vi "Verify Scroll.vi"(0 "GEA2 Reference In":refnum<k24>, 1 "Timeout (sec)":dbl, 2 "Scroll Text":string, 11 "Error In":errorcluster, 13 "Ignore Brightness?":bool) -> (4 "GEA2 Reference Out":refnum<k24>, 6 "Pass/Fail?":bool, 8 "Report Text":string, 15 "Error Out":errorcluster)   [LabVIEW 2016, in "TLMB.lvlib"]
doc: "This VI is used to verify SSD scrolling messages on the HEUI."
uses:
  Projects/TLMB.lvlib
  Q:/Common/DLLs/GEA3/GeaCommunication.dll
  Common/DLLs/GEA3/GeaCommunication.dll
  Common/LabVIEW GEA2 Toolkit/LabVIEW_GEA2_Toolkit.lvlibp/type defs/Source_Destination.ctl
  Common/LabVIEW GEA2 Toolkit/LabVIEW_GEA2_Toolkit.lvlibp/type defs/ERD Read Data In.ctl
  Common/LabVIEW GEA2 Toolkit/LabVIEW_GEA2_Toolkit.lvlibp/type defs/Data Type.ctl
  Common/LabVIEW GEA2 Toolkit/LabVIEW_GEA2_Toolkit.lvlibp
panel:
  in  "Standalone":bool
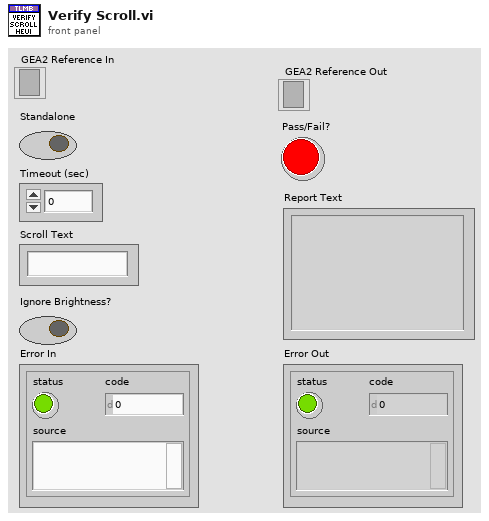
[diagram p1: front panel]
types:
  T1 = typedef "LabVIEW_GEA2_Toolkit.lvlibp/ERD Read Data In.ctl" = cluster{"ERD Number":u16, "Data Type":T2}
  T2 = typedef "LabVIEW_GEA2_Toolkit.lvlibp/Data Type.ctl" = enum16{"string", "boolean", "uint8_t", "uint16_t", "uint32_t", "uint64_t", "int8_t", "int16_t", "int32_t", "int64_t"}
  T3 = typedef "LabVIEW_GEA2_Toolkit.lvlibp/Source_Destination.ctl" = cluster{"Source":u8, "Destination":u8}
  T4 = typedef "TLMB.lvlib/HEUI_LEDs.ctl" = cluster{"Z101 - Start":bool, "Z103 - Colors":bool, "Z104 - Whites":bool, "Z105 - Towels":bool, "Z106 - Bulky Items":bool, "Z107 - Heavy Duty":bool, "Z108 - Jeans":bool, "Z109 - Basket Clean":bool, "Z110 - Drain and Spin":bool, "Z111 - Rinse and Spin":bool, "Z112 - Speed Wash":bool, "Z113 - Active Wear":bool, "Z114 - Hand Wash":bool, "Z115 - Delicates":bool, "Z116 - Easy Care":bool, "Z117 - Tomato":bool, "Z118 - Wine":bool, "Z119 - Blood":bool, "Z120 - Grass":bool, "Z121 - Dirt":bool, "Z122_MSB_A":bool, "Z123_MSB_B":bool, "Z124_MSB_G":bool, "Z125_MSB_C":bool, "Z126_MSB_D":bool, "Z127_MSB_E":bool, "Z128_MSB_F":bool, "Z129_LSB_A":bool, "Z130_LSB_B":bool, "Z131_LSB_G":bool, "Z132_LSB_C":bool, "Z133_LSB_D":bool, "Z134_LSB_E":bool, "Z135_LSB_F":bool, "Z136 - Pause":bool, "Z137 - Pause":bool, "Z138 - Lock Controls":bool, "Z139 - Lock Controls":bool, "Z140 - Lock Controls":bool, "Z141 - Lid Lock":bool, "Z142 - Lid Lock":bool, "Z143 - Lid Lock":bool, "Z144 - Good":bool, "Z145":bool, "Z146":bool, "Z147 - Better":bool, "Z148 - Delay":bool, "Z149 - Fill":bool, "Z150 - Soak":bool, "Z151 - Wash":bool, "Z152 - Rinse":bool, "Z153 - Spin":bool, "Z154 - Hot":bool, "Z155 - Warm":bool, "Z156 - Colors":bool, "Z157 - Cool":bool, "Z158 - Cold":bool, "Z159 - Tap Cold":bool, "Z160 - Extra Heavy":bool, "Z161 - Heavy":bool, "Z162 - Normal":bool, "Z163 - Light":bool, "Z164 - Max Spin":bool, "Z165 - More Spin":bool, "Z166 - Normal Spin":bool, "Z167 - No Spin":bool, "Z168 - Extra Rinse":bool, "Z170 - Deep Rinse":bool, "Z171 - Auto Soak":bool, "Z172 - Warm Rinse":bool, "Z173 - Deep Fill":bool, "Z174 - My Cycles":bool, "Z175 - Delay Wash":bool, "Z176 - Spin Stop":bool, "Z177 - Spin Stop":bool, "Z178 - Spin Stop":bool, "Z179 - Pause":bool, "Z109":bool, "Z110":bool, "Z123":bool, "Z124":bool, "Z140":bool, "Unused0":bool, "Unused1":bool, "Unused2":bool, "Unused3":bool, "Channel_Off":bool, "Channel_Cycle_Unmapped":bool}
  T5 = typedef "TLMB.lvlib/HEUI_Display.ctl" = cluster{"SSD":string, "Cycle Selection":T6, "Stain Selection":T7, "Temp Level":T8, "Soil Level":T9, "Spin Level":T10, "750 Status":T11, "Start":bool, "Pause/WiFi":bool, "Lock Controls":bool, "Lid Lock":bool, "Extra Rinse":bool, "Deep Rinse":bool, "Auto Soak":bool, "Warm Rinse":bool, "Deep Fill":bool, "My Cycle":bool, "Delay Wash":bool, "Spin Stop":bool, "Delay":bool, "Fill":bool, "Soak":bool, "Wash":bool, "Rinse":bool, "Spin":bool}
  T6 = typedef "TLMB.lvlib/Cycle Selection Enum.ctl" = enum16{"Colors", "Easy Care", "Delicates", "Hand Wash", "Active Wear", "Speed Wash", "Rinse and Spin", "Drain and Spin", "Basket Clean", "Jeans", "Heavy Duty", "Bulky Items", "Towels", "Whites", "Off", "*Incorrect*"}
  T7 = typedef "TLMB.lvlib/Stain Enum.ctl" = enum16{"Tomato", "Wine", "Blood", "Grass", "Dirt", "Off", "*Incorrect*"}
  T8 = typedef "TLMB.lvlib/Temp Enum.ctl" = enum16{"Hot", "Warm", "Colors", "Cool", "Cold", "Tap Cold", "Off", "*Incorrect*"}
  T9 = typedef "TLMB.lvlib/Soil Enum.ctl" = enum16{"Extra Heavy", "Heavy", "Normal", "Light", "Off", "*Incorrect*"}
  T10 = typedef "TLMB.lvlib/Spin Enum.ctl" = enum16{"Max Spin", "More Spin", "Normal Spin", "No Spin", "Off", "*Incorrect*"}
  T11 = typedef "TLMB.lvlib/750 Status Enum.ctl" = enum16{"Fill", "Wash", "Rinse", "Spin", "Off", "*Incorrect*"}
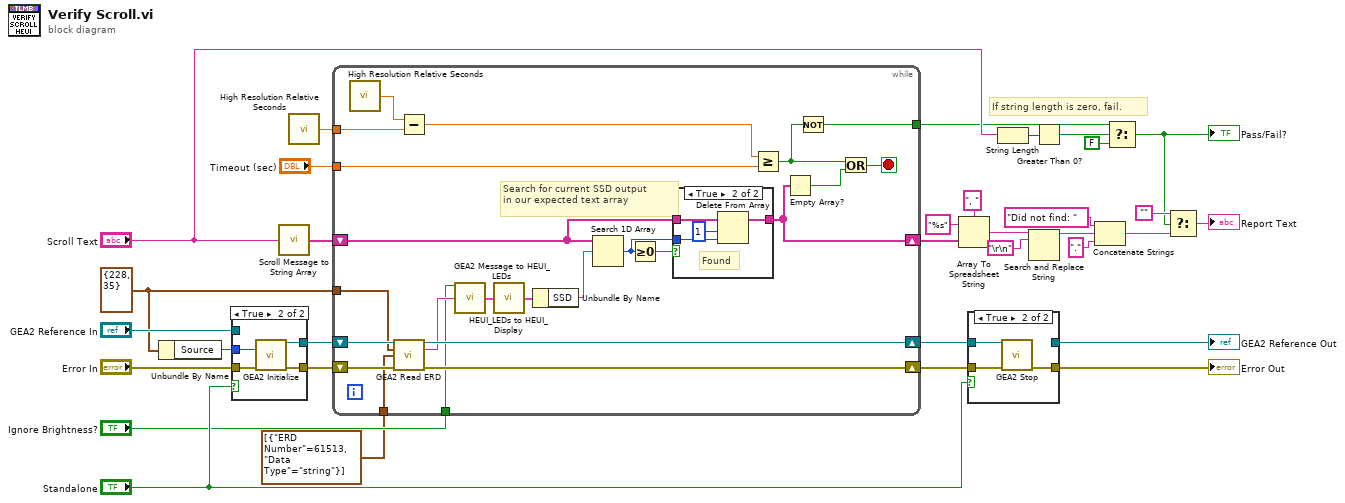
[diagram p0: block diagram]
diagram:
  w20 = T3 {"Source"=228, "Destination"=35} ("GEA Inputs")
  # "If string length is zero, fail."
  n1 = Unbundle By Name(w20) -> ("Source"=w32:u8)
  n2 = case shown="True" "Standalone" {
    tunnel: "Error In" -> [w35 w39]
    tunnel: w32 -> [_ w38]
    tunnel: [w34 w37] -> w28
    tunnel: [w35 w36] -> w27
    tunnel: "GEA2 Reference In" -> [w34 _]
    frame False {
    }
    frame True {
      n3 = call "GEA2 Initialize.vi"("Source Address"=w38, "error in"=w39) -> ("GEA2 Reference Out"=w37:refnum<k24>, "error out"=w36:errorcluster)  [unwired: 11 in, 1 out]
    }
  }
  n4 = call "Scroll Message to String Array.vi"("Scroll Text"="Scroll Text") -> ("Array"=w23:string[])  [unwired: 14 in]
  n5 = call <vilib>:"High Resolution Relative Seconds.vi"() -> ("relative seconds"=w21:dbl)
  n6 = while {
    tunnel: w21 -> [w61]
    tunnel: [w41] -> w2
    tunnel: "Ignore Brightness?" -> [w51]
    shift-right: [w57] -> w26
    shift-left: w28 -> [w54]
    shift-right: [w56] -> w25
    shift-left: w27 -> [w55]
    tunnel: T1[] [{"ERD Number"=61513, "Data Type"=enum."string"}] ("Read ERD List") -> [w53]
    shift-right: [w40] -> w16
    shift-left: w23 -> [w45]
    tunnel: w20 -> [w43]
    tunnel: "Timeout (sec)" -> [w42]
    stop <- w59 stop-if-true
    # "Search for current SSD output\nin our expected text array"
    n7 = call <vilib>:"High Resolution Relative Seconds.vi"() -> ("relative seconds"=w62:dbl)
    n8 = call "GEA2 Read ERD.vi"("GEA2 Reference In"=w54, "GEA Inputs"=w43, "Read ERD List"=w53, "Error In"=w55) -> ("GEA2 Reference Out"=w57:refnum<k24>, "Raw Data Out"=w52:string, "Error Out"=w56:errorcluster)  [unwired: 8 in, 1 out]
    n9 = Subtract(x=w62, y=w61) -> (x-y=w60:dbl)
    n10 = call "GEA2 Message to HEUI_LEDs.vi"("Ignore Brightness?"=w51, "Raw Data In"=w52) -> ("HEUI_LEDs"=w50:T4)  [unwired: 13 in]
    n11 = call "HEUI_LEDs to HEUI_Display.vi"("HEUI_LEDs"=w50) -> ("HEUI_Display"=w49:T5)  [unwired: 14 in]
    n12 = Unbundle By Name(w49) -> ("SSD"=w48:string)
    n13 = Search 1D Array(1D array=w45, element=w48) -> (index of element=w46:i32)  [unwired: 1 in]
    n14 = Greater Or Equal To 0?(x=w46) -> (x >= 0?=w47:bool)
    n15 = case shown="True" w47 {
      tunnel: w46 -> [_ w66]
      tunnel: w45 -> [w63 w67]
      tunnel: [w63 w64] -> w40
      frame False {
        # "Not Found"
      }
      frame True {
        # "Found"
        n16 = Delete From Array(array=w67, length=1, index=w66) -> (array with subset deleted=w64:string[])  [unwired: 1 out]
      }
    }
    n17 = Greater Or Equal?(x=w60, y=w42) -> (x >= y?=w58:bool)
    n18 = Empty Array?(array=w40) -> (empty?=w44:bool)
    n19 = Not(x=w58) -> (.not. x?=w41:bool)
    n20 = Or(x=w58, y=w44) -> (x .or. y?=w59:bool)
  }
  n21 = Array To Spreadsheet String(delimiter (Tab)=", ", array=w16, 3:"%s" ("format string")) -> (spreadsheet string=w10:string)
  n22 = case shown="True" "Standalone" {
    tunnel: w25 -> [w69 w72]
    tunnel: [w69 w71] -> w12
    tunnel: w26 -> [w68 w70]
    tunnel: [w68 _] -> w29
    frame False {
    }
    frame True {
      n23 = call "GEA2 Stop.vi"("GEA2 Reference In"=w70, "Error In"=w72) -> ("Error Out"=w71:errorcluster)  [unwired: 13 in]
    }
  }
  "GEA2 Reference Out" <- w29
  "Error Out" <- w12
  n24 = String Length(string="Scroll Text") -> (length=w5:i32)
  n25 = Search and Replace String(input string=w10, search string="\r\n") -> (result string=w8:string)  [unwired: 6 in, 3 out]
  n26 = Greater Than 0?(x=w5) -> (x > 0?=w4:bool)
  n27 = Concatenate Strings("Did not find: " ("string"), w8, "." ("string")) -> (w7:string)
  n28 = Select(t=w2, s=w4, f=FALSE) -> (s? t:f=w3:bool)
  "Pass/Fail?" <- w3
  n29 = Select(t="", s=w3, f=w7) -> (s? t:f=→"Report Text":string)
